vi "Get Border Rect.vi"(8 "error in (no error)":errorcluster caption="Error in (no error)", 11 "borderObj Ref":refnum<vi>) -> (0 "error out":errorcluster, 3 "Rect":T1)   [LabVIEW 2017]
doc: "Follows the decorations around the object wired to borderObj Ref and returns the rectangle they enclose."
uses:
  <vilib>/Utility/miscctls.llb/LVRectTypeDef.ctl
  _openG/_reuse_openG.lvlib
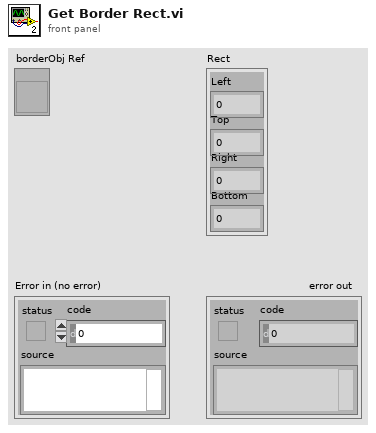
[diagram p1: front panel]
types:
  T1 = typedef "LVRectTypeDef.ctl" = cluster{"Left":i16, "Top":i16, "Right":i16, "Bottom":i16}
  T2 = typedef "LVPointTypeDef.ctl" = cluster{"Horizontal":i16, "Vertical":i16}
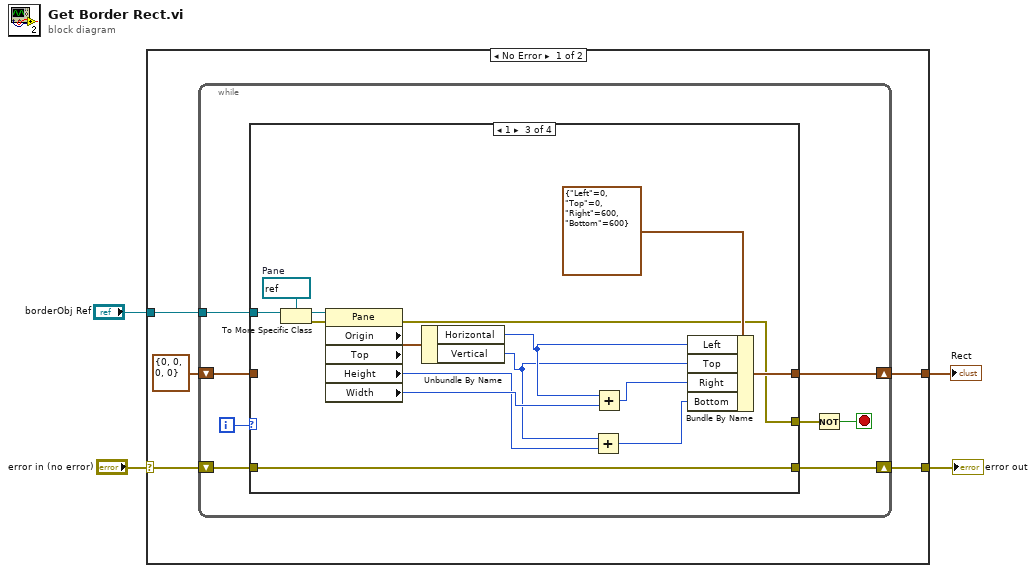
[diagram p0: block diagram]
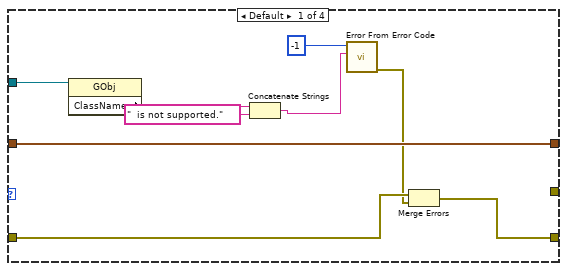
[diagram p2: hidden frame]
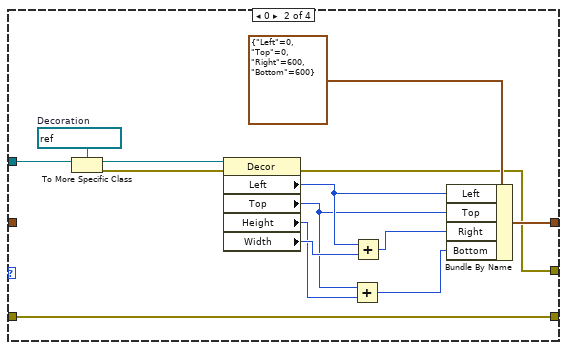
[diagram p3: hidden frame]
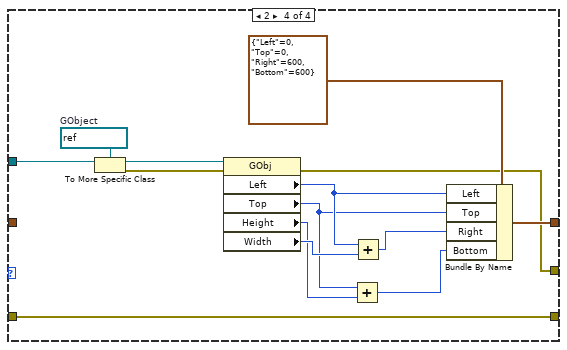
[diagram p4: hidden frame]
diagram:
  n1 = case shown="No Error" "error in (no error)" {
    selector: "error in (no error)" -> [w5 w70]
    tunnel: [w9 _] -> w4
    tunnel: "borderObj Ref" -> [w8 _]
    tunnel: [w6 w70] -> w2
    frame No Error {
      n2 = while {
        tunnel: w8 -> [w17]
        shift-right: [w16] -> w9
        shift-left: T1 {"Left"=0, "Top"=0, "Right"=0, "Bottom"=0} ("Rect") -> [w13]
        shift-right: [w11] -> w6
        shift-left: w5 -> [w10]
        i -> [w15]
        stop <- w12 stop-if-true
        n3 = case shown="1" w15 {
          tunnel: w17 -> [w21 w40 w55 w69]
          tunnel: [w26 w32 w49 w61] -> w16
          tunnel: [_ w28 w45 w57] -> w14
          tunnel: w13 -> [w26 _ _ _]
          tunnel: [w24 w27 w41 w56] -> w11
          tunnel: w10 -> [w25 w27 w41 w56]
          frame Default {
            n4 = property class="GObj"(reference=w21) -> ("ClassName"=w20:string)  [unwired: 1 in, 2 out]
            n5 = Concatenate Strings(w20, "  is not supported." ("string")) -> (w18:string)
            n6 = call "Error From Error Code.vi"("error message (\"\")"=w18, "error code (0)"=-1) -> ("error out"=w22:errorcluster)  [unwired: 7 in]
            n7 = Merge Errors(w25, w22) -> (w24:errorcluster)
          }
          frame 0 {
            w30 = refnum<vi> refnum  # Decoration
            n8 = To More Specific Class(target class=w30, reference=w40) -> (specific class reference=w31:refnum<vi>, error out=w29:errorcluster)  [unwired: 1 in]
            n9 = property class="Decor"(reference=w31, error in=w29) -> (error out=w28:errorcluster, "Left"=w36:i32, "Top"=w35:i32, "Height"=w38:u32, "Width"=w39:u32)  [unwired: 1 out]
            n10 = Add(x=w35, y=w38) -> (x+y=w33:u32)
            n11 = Add(x=w36, y=w39) -> (x+y=w34:u32)
            n12 = Bundle By Name(cluster=T1 {"Left"=0, "Top"=0, "Right"=600, "Bottom"=600} ("Rect"), "Left"=w36, "Top"=w35, "Right"=w34, "Bottom"=w33) -> (w32:T1)
          }
          frame 1 {
            w47 = refnum<vi> refnum  # Pane
            n13 = To More Specific Class(target class=w47, reference=w55) -> (specific class reference=w48:refnum<vi>, error out=w46:errorcluster)  [unwired: 1 in]
            n14 = property class="Pane" props=["Origin", "Top", "Height", "Width"](reference=w48, error in=w46) -> (error out=w45:errorcluster, "Origin"=w44:T2, "Height"=w53:u32, "Width"=w54:u32)  [unwired: 2 out]
            n15 = Unbundle By Name(w44) -> ("Horizontal"=w43:i16, "Vertical"=w42:i16)
            n16 = Add(x=w42, y=w53) -> (x+y=w50:u32)
            n17 = Add(x=w43, y=w54) -> (x+y=w51:u32)
            n18 = Bundle By Name(cluster=T1 {"Left"=0, "Top"=0, "Right"=600, "Bottom"=600} ("Rect"), "Left"=w43, "Top"=w42, "Right"=w51, "Bottom"=w50) -> (w49:T1)
          }
          frame 2 {
            w59 = refnum<vi> refnum  # GObject
            n19 = To More Specific Class(target class=w59, reference=w69) -> (specific class reference=w60:refnum<vi>, error out=w58:errorcluster)  [unwired: 1 in]
            n20 = property class="GObj"(reference=w60, error in=w58) -> (error out=w57:errorcluster, "Left"=w65:i32, "Top"=w64:i32, "Height"=w67:u32, "Width"=w68:u32)  [unwired: 1 out]
            n21 = Add(x=w64, y=w67) -> (x+y=w62:u32)
            n22 = Add(x=w65, y=w68) -> (x+y=w63:u32)
            n23 = Bundle By Name(cluster=T1 {"Left"=0, "Top"=0, "Right"=600, "Bottom"=600} ("Rect"), "Left"=w65, "Top"=w64, "Right"=w63, "Bottom"=w62) -> (w61:T1)
          }
        }
        n24 = Not(x=w14) -> (.not. x?=w12:bool)
      }
    }
    frame Error {
    }
  }
  "Rect" <- w4
  "error out" <- w2
